vi "Decode Message.vi"(11 "Message":u8[](array[numeric]) format="%.0x") -> (0 "Range (0..6)":i32, 1 "Function (0..15)":T1, 2 "Value":dbl, 3 "Display string":string, 4 "State 1":enum16{"OFF", "AC", "DC", "AC+DC"}(ring), 6 "State 2":enum16{"OFF", "Auto", "Manual", "Undefined"}(ring))   [LabVIEW 2015, in "VC940.lvlib"]
uses:
  VC940.lvlib
  Controls/Function.ctl
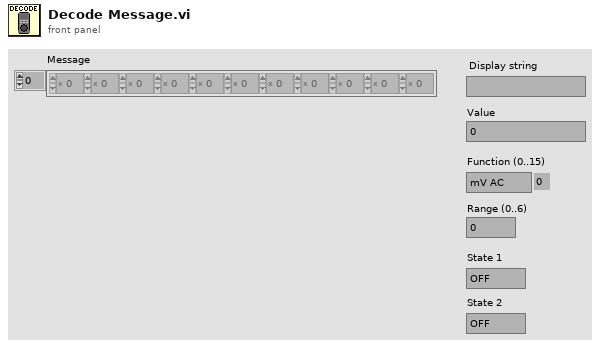
[diagram p1: front panel]
types:
  T1 = typedef "VC940.lvlib/Function.ctl" = enum8{"mV AC", "V DC", "V AC", "mV DC", "Ohm", "nF", "°C", "µA", "mA", "A", "Ohm Fm", "V Diode", "Hz", "°F", "W", "%4-20mA"}
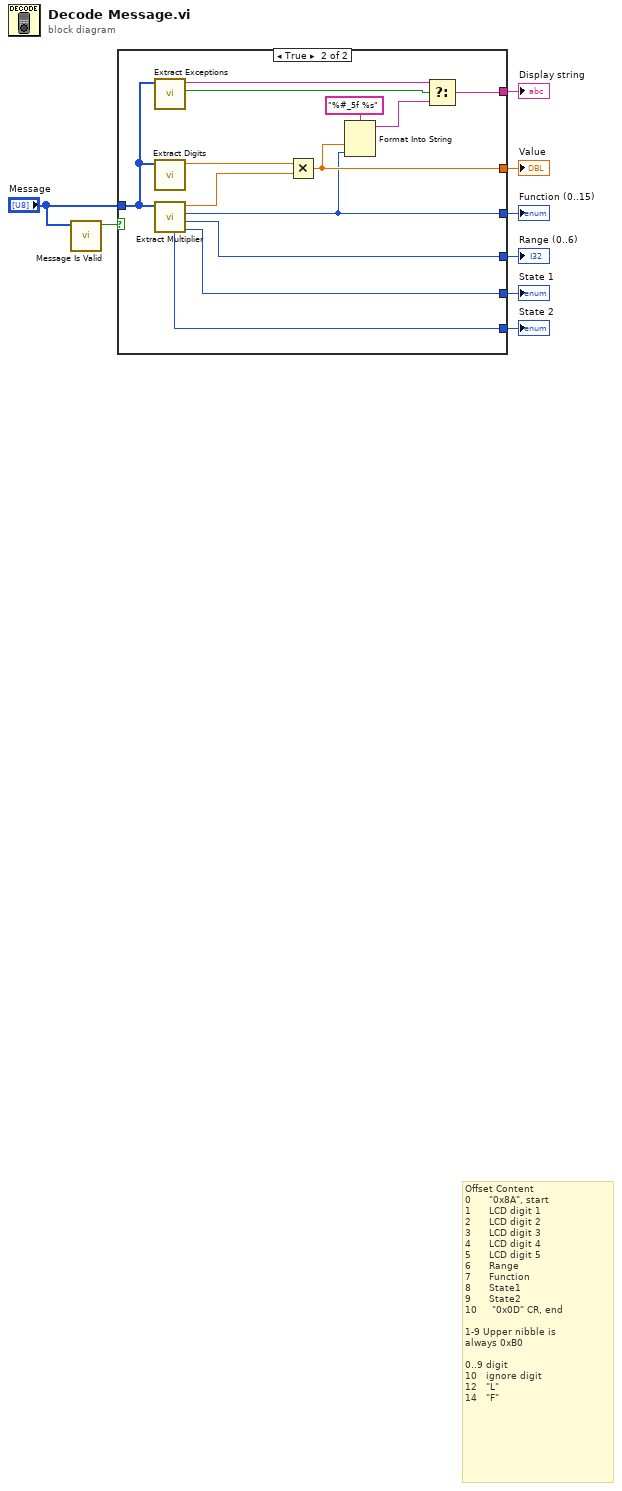
[diagram p0: block diagram]
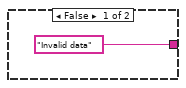
[diagram p2: hidden frame]
diagram:
  # "Offset Content\n0      \"0x8A\", start\n1      LCD digit 1\n2      LCD digit 2\n3      LCD digit 3\n4      LCD digit 4\n5      LCD digit 5\n6      Range\n7      Function\n8      State1\n9      State2\n10     \"0x0D\" CR, end\n\n1-9 Upper nibble is\nalways 0xB0\n\n0..9 digit\n10   ignore digit\n12   \"L\"\n14   \"F\""
  n1 = call "Message Is Valid.vi"("Message"="Message") -> ("Valid"=w8:bool)  [unwired: 10 in]
  n2 = case shown="True" w8 {
    tunnel: [_ w16] -> w4
    tunnel: "Message" -> [_ w14]
    tunnel: [_ w22] -> w5
    tunnel: [_ w21] -> w6
    tunnel: [_ w20] -> w7
    tunnel: [_ w17] -> w3
    tunnel: ["Invalid data" ("Display string") w10] -> w1
    frame False {
    }
    frame True {
      n3 = call "Extract Exceptions.vi"("Message"=w14) -> ("Exception"=w12:bool, "Display string"=w11:string)  [unwired: 9 in]
      n4 = call "Extract Digits.vi"("Message"=w14) -> ("DMM digits"=w15:dbl)  [unwired: 9 in, 1 out]
      n5 = call "Extract Multiplier.vi"("Message"=w14) -> ("State 1"=w21:enum16{"OFF", "AC", "DC", "AC+DC"}, "Range (0..6)"=w22:i32, "Function (0..15)"=w16:T1, "Multiplier"=w19:dbl, "State 2"=w20:enum16{"OFF", "Auto", "Manual", "Undefined"})  [unwired: 6 in]
      n6 = Multiply(x=w15, y=w19) -> (x*y=w17:dbl)
      n7 = Format Into String(format string="%#_5f %s", w17, w16) -> (resulting string=w13:string)  [unwired: 2 in, 1 out]
      n8 = Select(t=w11, s=w12, f=w13) -> (s? t:f=w10:string)
    }
  }
  "Function (0..15)" <- w4
  "Range (0..6)" <- w5
  "State 1" <- w6
  "State 2" <- w7
  "Value" <- w3
  "Display string" <- w1
